vi "test-rotation2d.vi"(8 "error in (no error)":errorcluster) -> (0 "error out":errorcluster, 3 "ALL TESTS PASSED":bool)   [LabVIEW 2019]
uses:
  <vilib>/Rock Robotics/WPI/ThirdParty/JAS_Junk/TrajLib/Util_CalcDist.vi
  <vilib>/Rock Robotics/WPI/ThirdParty/JAS_Junk/TrajLib/Rotation_UnaryMinus.vi
  <vilib>/Rock Robotics/WPI/ThirdParty/JAS_Junk/TrajLib/Rotation_CreateXY.vi
  <vilib>/Rock Robotics/WPI/ThirdParty/JAS_Junk/TrajLib/Trajectory_Library.lvlib
panel:
  out "T7 - True":bool
  out "T4 -- X -- 0":dbl
  out "T3 -- X -- 0":dbl
  out "T2 -- y -- 0":dbl
  out "T2 -- X -- 0":dbl
  out "T6 - False":bool
  out "T5 - True":bool
  out "T1 -- y -- 0":dbl
  out "T1 -- X -- 0":dbl
  out "T0 -- y -- 0":dbl
  out "T0 -- X -- 0":dbl
  # "Rotation2D Test"
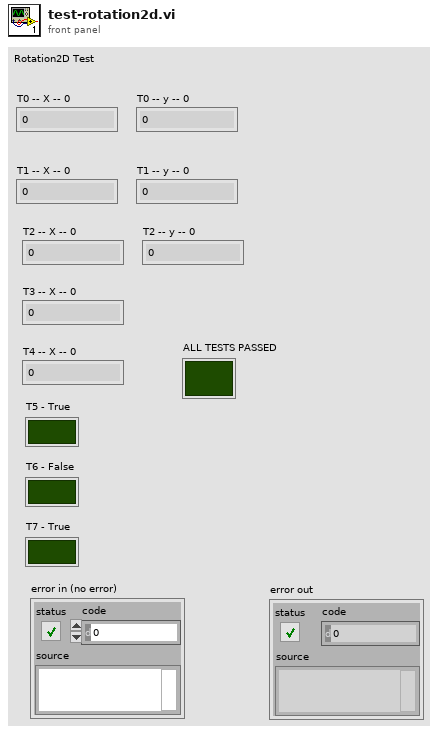
[diagram p1: front panel]
types:
  T1 = typedef "Trajectory_Library.lvlib/ROTATION2D.ctl" = cluster{"VALUE":dbl, "COS":dbl, "SIN":dbl}
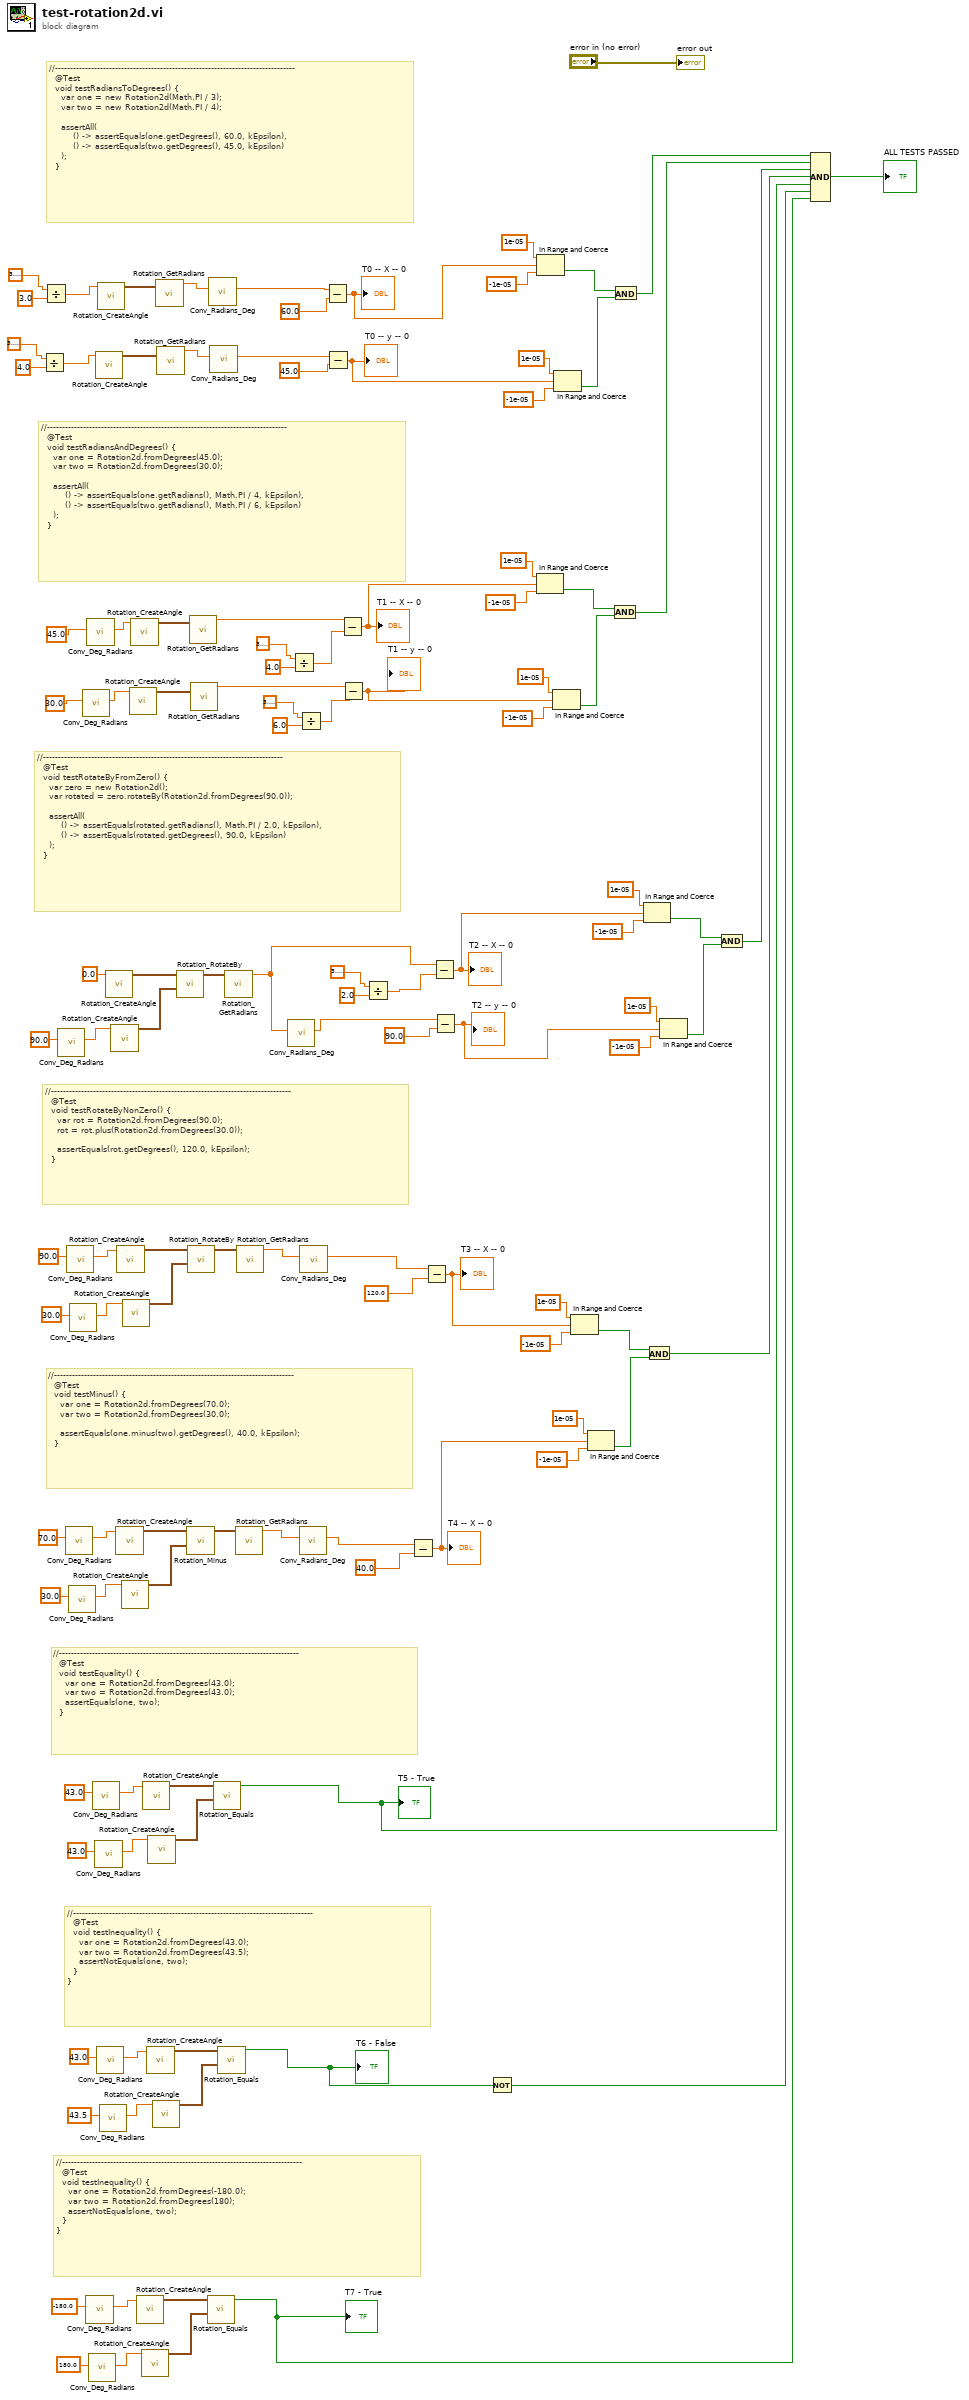
[diagram p0: block diagram]
diagram:
  # "//--------------------------------------------------------------------------------\n  @Test\n  void testInequality() {\n    var one = Rotation2d.fromDegrees(-180.0);\n    var two = Rotation2d.fromDegrees(180);\n    assertNotEquals(one, two);\n  }\n}"
  # "//--------------------------------------------------------------------------------\n  @Test\n  void testInequality() {\n    var one = Rotation2d.fromDegrees(43.0);\n    var two = Rotation2d.fromDegrees(43.5);\n    assertNotEquals(one, two);\n  }\n}"
  # "//--------------------------------------------------------------------------------\n  @Test\n  void testMinus() {\n    var one = Rotation2d.fromDegrees(70.0);\n    var two = Rotation2d.fromDegrees(30.0);\n\n    assertEquals(one.minus(two).getDegrees(), 40.0, kEpsilon);\n  }"
  # "//--------------------------------------------------------------------------------\n  @Test\n  void testRotateByNonZero() {\n    var rot = Rotation2d.fromDegrees(90.0);\n    rot = rot.plus(Rotation2d.fromDegrees(30.0));\n\n    assertEquals(rot.getDegrees(), 120.0, kEpsilon);\n  }"
  # "//--------------------------------------------------------------------------------\n  @Test\n  void testRotateByFromZero() {\n    var zero = new Rotation2d();\n    var rotated = zero.rotateBy(Rotation2d.fromDegrees(90.0));\n\n    assertAll(\n        () -> assertEquals(rotated.getRadians(), Math.PI / 2.0, kEpsilon),\n        () -> assertEquals(rotated.getDegrees(), 90.0, kEpsilon)\n    );\n  }"
  # "//--------------------------------------------------------------------------------\n  @Test\n  void testEquality() {\n    var one = Rotation2d.fromDegrees(43.0);\n    var two = Rotation2d.fromDegrees(43.0);\n    assertEquals(one, two);\n  }"
  # "//--------------------------------------------------------------------------------\n  @Test\n  void testRadiansAndDegrees() {\n    var one = Rotation2d.fromDegrees(45.0);\n    var two = Rotation2d.fromDegrees(30.0);\n\n    assertAll(\n        () -> assertEquals(one.getRadians(), Math.PI / 4, kEpsilon),\n        () -> assertEquals(two.getRadians(), Math.PI / 6, kEpsilon)\n    );\n  }"
  # "//--------------------------------------------------------------------------------\n  @Test\n  void testRadiansToDegrees() {\n    var one = new Rotation2d(Math.PI / 3);\n    var two = new Rotation2d(Math.PI / 4);\n\n    assertAll(\n        () -> assertEquals(one.getDegrees(), 60.0, kEpsilon),\n        () -> assertEquals(two.getDegrees(), 45.0, kEpsilon)\n    );\n  }"
  n1 = Divide(x=3.141592653589793, y=4.0) -> (x/y=w108:dbl)
  n2 = Divide(x=3.141592653589793, y=3.0) -> (x/y=w111:dbl)
  n3 = call <vilib>:"Conv_Deg_Radians.vi"("Degress"=90.0) -> ("Radians"=w117:dbl)  [unwired: 10 in]
  n4 = call <vilib>:"Conv_Deg_Radians.vi"("Degress"=70.0) -> ("Radians"=w62:dbl)  [unwired: 10 in]
  n5 = call <vilib>:"Conv_Deg_Radians.vi"("Degress"=90.0) -> ("Radians"=w71:dbl)  [unwired: 10 in]
  n6 = call <vilib>:"Conv_Deg_Radians.vi"("Degress"=30.0) -> ("Radians"=w69:dbl)  [unwired: 10 in]
  n7 = call <vilib>:"Conv_Deg_Radians.vi"("Degress"=30.0) -> ("Radians"=w78:dbl)  [unwired: 10 in]
  n8 = call <vilib>:"Conv_Deg_Radians.vi"("Degress"=30.0 ("y")) -> ("Radians"=w93:dbl)  [unwired: 10 in]
  n9 = call <vilib>:"Conv_Deg_Radians.vi"("Degress"=-180.0) -> ("Radians"=w43:dbl)  [unwired: 10 in]
  n10 = call <vilib>:"Conv_Deg_Radians.vi"("Degress"=45.0 ("y")) -> ("Radians"=w92:dbl)  [unwired: 10 in]
  n11 = call <vilib>:"Conv_Deg_Radians.vi"("Degress"=180.0) -> ("Radians"=w48:dbl)  [unwired: 10 in]
  n12 = call <vilib>:"Conv_Deg_Radians.vi"("Degress"=43.0) -> ("Radians"=w55:dbl)  [unwired: 10 in]
  n13 = call <vilib>:"Conv_Deg_Radians.vi"("Degress"=43.0) -> ("Radians"=w60:dbl)  [unwired: 10 in]
  n14 = call <vilib>:"Rotation_CreateAngle.vi"("Angle"=w108) -> ("ROTATION"=w104:T1)  [unwired: 10 in]
  n15 = call <vilib>:"Conv_Deg_Radians.vi"("Degress"=43.0) -> ("Radians"=w49:dbl)  [unwired: 10 in]
  n16 = call <vilib>:"Rotation_CreateAngle.vi"("Angle"=w111) -> ("ROTATION"=w107:T1)  [unwired: 10 in]
  n17 = call <vilib>:"Conv_Deg_Radians.vi"("Degress"=43.5) -> ("Radians"=w54:dbl)  [unwired: 10 in]
  n18 = call <vilib>:"Rotation_CreateAngle.vi"("Angle"=0.0) -> ("ROTATION"=w86:T1)  [unwired: 10 in]
  n19 = call <vilib>:"Rotation_CreateAngle.vi"("Angle"=w117) -> ("ROTATION"=w85:T1)  [unwired: 10 in]
  n20 = call <vilib>:"Rotation_CreateAngle.vi"("Angle"=w62) -> ("ROTATION"=w67:T1)  [unwired: 10 in]
  n21 = call <vilib>:"Rotation_CreateAngle.vi"("Angle"=w71) -> ("ROTATION"=w76:T1)  [unwired: 10 in]
  n22 = call <vilib>:"Rotation_CreateAngle.vi"("Angle"=w69) -> ("ROTATION"=w66:T1)  [unwired: 10 in]
  n23 = call <vilib>:"Rotation_CreateAngle.vi"("Angle"=w78) -> ("ROTATION"=w75:T1)  [unwired: 10 in]
  n24 = call <vilib>:"Rotation_CreateAngle.vi"("Angle"=w93) -> ("ROTATION"=w100:T1)  [unwired: 10 in]
  n25 = call <vilib>:"Rotation_CreateAngle.vi"("Angle"=w92) -> ("ROTATION"=w101:T1)  [unwired: 10 in]
  n26 = call <vilib>:"Rotation_CreateAngle.vi"("Angle"=w43) -> ("ROTATION"=w46:T1)  [unwired: 10 in]
  n27 = call <vilib>:"Rotation_CreateAngle.vi"("Angle"=w48) -> ("ROTATION"=w45:T1)  [unwired: 10 in]
  n28 = call <vilib>:"Rotation_CreateAngle.vi"("Angle"=w55) -> ("ROTATION"=w58:T1)  [unwired: 10 in]
  n29 = call <vilib>:"Rotation_CreateAngle.vi"("Angle"=w49) -> ("ROTATION"=w52:T1)  [unwired: 10 in]
  n30 = call <vilib>:"Rotation_CreateAngle.vi"("Angle"=w60) -> ("ROTATION"=w57:T1)  [unwired: 10 in]
  n31 = call <vilib>:"Rotation_CreateAngle.vi"("Angle"=w54) -> ("ROTATION"=w51:T1)  [unwired: 10 in]
  n32 = call <vilib>:"Rotation_GetRadians.vi"("in ROTATION"=w107) -> ("AngleRadians"=w106:dbl)  [unwired: 10 in]
  n33 = call <vilib>:"Rotation_GetRadians.vi"("in ROTATION"=w104) -> ("AngleRadians"=w105:dbl)  [unwired: 10 in]
  n34 = call <vilib>:"Rotation_RotateBy.vi"("other Rotation"=w85, "in ROTATION"=w86) -> ("out ROTATION"=w84:T1)  [unwired: 9 in]
  n35 = call <vilib>:"Rotation_Minus.vi"("other ROTATION"=w66, "in ROTATION"=w67) -> ("out ROTATION"=w65:T1)  [unwired: 9 in]
  n36 = call <vilib>:"Rotation_RotateBy.vi"("other Rotation"=w75, "in ROTATION"=w76) -> ("out ROTATION"=w74:T1)  [unwired: 9 in]
  n37 = call <vilib>:"Rotation_GetRadians.vi"("in ROTATION"=w101) -> ("AngleRadians"=w89:dbl)  [unwired: 10 in]
  n38 = call <vilib>:"Rotation_GetRadians.vi"("in ROTATION"=w100) -> ("AngleRadians"=w88:dbl)  [unwired: 10 in]
  n39 = call <vilib>:"Rotation_Equals.vi"("other ROTATION"=w45, "in ROTATION"=w46) -> ("Equals"=w2:bool)  [unwired: 9 in]
  "T7 - True" <- w2
  n40 = call <vilib>:"Conv_Radians_Deg.vi"("Radians"=w106) -> ("Degrees"=w103:dbl)  [unwired: 10 in]
  n41 = call <vilib>:"Conv_Radians_Deg.vi"("Radians"=w105) -> ("Degrees"=w102:dbl)  [unwired: 10 in]
  n42 = call <vilib>:"Rotation_Equals.vi"("other ROTATION"=w57, "in ROTATION"=w58) -> ("Equals"=w4:bool)  [unwired: 9 in]
  "T5 - True" <- w4
  n43 = call <vilib>:"Rotation_Equals.vi"("other ROTATION"=w51, "in ROTATION"=w52) -> ("Equals"=w5:bool)  [unwired: 9 in]
  "T6 - False" <- w5
  n44 = call <vilib>:"Rotation_GetRadians.vi"("in ROTATION"=w84) -> ("AngleRadians"=w80:dbl)  [unwired: 10 in]
  n45 = call <vilib>:"Rotation_GetRadians.vi"("in ROTATION"=w65) -> ("AngleRadians"=w64:dbl)  [unwired: 10 in]
  n46 = call <vilib>:"Rotation_GetRadians.vi"("in ROTATION"=w74) -> ("AngleRadians"=w73:dbl)  [unwired: 10 in]
  n47 = call <vilib>:"Conv_Radians_Deg.vi"("Radians"=w80) -> ("Degrees"=w79:dbl)  [unwired: 10 in]
  n48 = Divide(x=3.141592653589793, y=4.0) -> (x/y=w94:dbl)
  n49 = Divide(x=3.141592653589793, y=6.0) -> (x/y=w95:dbl)
  n50 = call <vilib>:"Conv_Radians_Deg.vi"("Radians"=w64) -> ("Degrees"=w61:dbl)  [unwired: 10 in]
  n51 = call <vilib>:"Conv_Radians_Deg.vi"("Radians"=w73) -> ("Degrees"=w70:dbl)  [unwired: 10 in]
  n52 = Subtract(x=w103, y=60.0) -> (x-y=w36:dbl)
  "T0 -- X -- 0" <- w36
  n53 = Subtract(x=w102, y=45.0) -> (x-y=w35:dbl)
  "T0 -- y -- 0" <- w35
  n54 = Subtract(x=w89, y=w94) -> (x-y=w25:dbl)
  "T1 -- X -- 0" <- w25
  n55 = Subtract(x=w88, y=w95) -> (x-y=w26:dbl)
  "T1 -- y -- 0" <- w26
  n56 = Divide(x=3.141592653589793, y=2.0) -> (x/y=w81:dbl)
  n57 = Subtract(x=w61, y=40.0 ("x")) -> (x-y=w7:dbl)
  "T4 -- X -- 0" <- w7
  n58 = Subtract(x=w70, y=120.0 ("x")) -> (x-y=w8:dbl)
  "T3 -- X -- 0" <- w8
  n59 = Subtract(x=w80, y=w81) -> (x-y=w17:dbl)
  "T2 -- X -- 0" <- w17
  n60 = Subtract(x=w79, y=90.0) -> (x-y=w16:dbl)
  "T2 -- y -- 0" <- w16
  n61 = Not(x=w5) -> (.not. x?=w3:bool)
  n62 = In Range and Coerce(upper limit=1e-05, x=w25, lower limit=-1e-05) -> (In Range?=w28:bool)  [unwired: 1 out]
  n63 = In Range and Coerce(upper limit=1e-05, x=w36, lower limit=-1e-05) -> (In Range?=w38:bool)  [unwired: 1 out]
  n64 = In Range and Coerce(upper limit=1e-05, x=w26, lower limit=-1e-05) -> (In Range?=w27:bool)  [unwired: 1 out]
  n65 = In Range and Coerce(upper limit=1e-05, x=w35, lower limit=-1e-05) -> (In Range?=w37:bool)  [unwired: 1 out]
  n66 = In Range and Coerce(upper limit=1e-05, x=w8, lower limit=-1e-05) -> (In Range?=w10:bool)  [unwired: 1 out]
  n67 = In Range and Coerce(upper limit=1e-05, x=w7, lower limit=-1e-05) -> (In Range?=w9:bool)  [unwired: 1 out]
  n68 = And(x=w28, y=w27) -> (x .and. y?=w24:bool)
  n69 = And(x=w38, y=w37) -> (x .and. y?=w33:bool)
  n70 = In Range and Coerce(upper limit=1e-05, x=w17, lower limit=-1e-05) -> (In Range?=w19:bool)  [unwired: 1 out]
  n71 = And(x=w10, y=w9) -> (x .and. y?=w6:bool)
  n72 = In Range and Coerce(upper limit=1e-05, x=w16, lower limit=-1e-05) -> (In Range?=w18:bool)  [unwired: 1 out]
  n73 = And(x=w19, y=w18) -> (x .and. y?=w15:bool)
  n74 = Compound Arithmetic op=AND(w33, w24, w15, w6, w4, w3, w2) -> (→"ALL TESTS PASSED":bool)
  "error out" <- "error in (no error)"
